vi "plot_functions.vi"() -> ()   [LabVIEW 2013]
doc: "opens a plot window and can access all the plot functions for testing"
uses:
  Classes/StatusLog/StatusLog.lvclass
  Classes/Plots/Plots.lvclass
  global variables.vi
  <vilib>/Utility/file.llb/Read From Spreadsheet File (string).vi
  MSEval/global_variables.vi
panel:
  in  "Combo Box":string(combo)="linear"
  in  "fit button":bool
  in  "data file":path=path "C:/Users/Thermo/Documents/GitHub/HelixMC/MSControl/test_vis/plot_data_he3.txt"
  in  "plot dataset button":bool
  in  "open plot button":bool
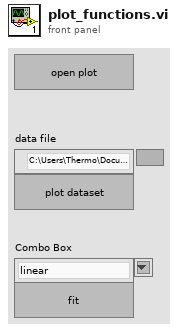
[diagram p1: front panel]
types:
  T1 = cluster{"log identifier":string, "active?":bool}[]
  T2 = cluster{"format string":string, "Variant":variant}
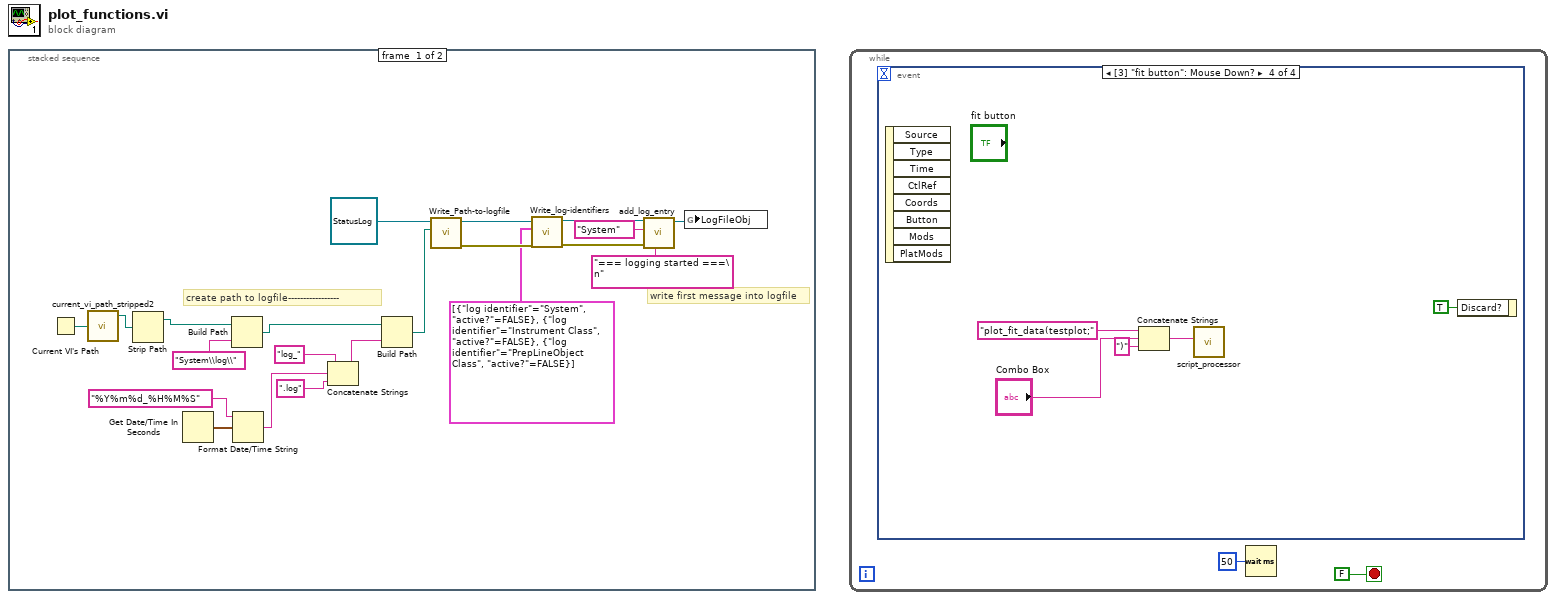
[diagram p0: block diagram]
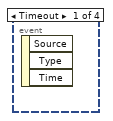
[diagram p2: hidden frame]
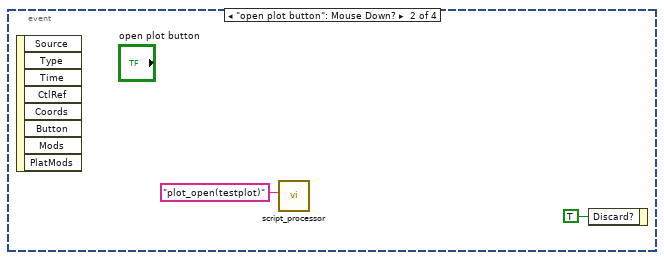
[diagram p3: hidden frame]
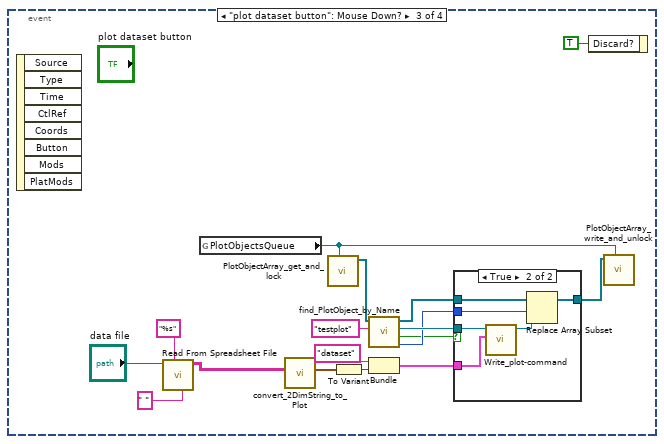
[diagram p4: hidden frame]
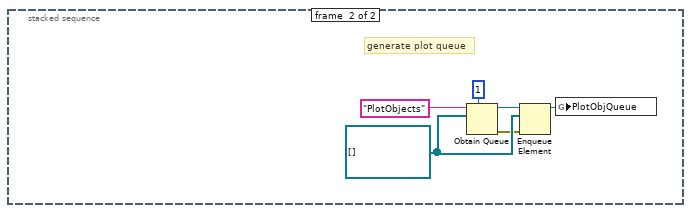
[diagram p6: hidden frame]
diagram:
  n1 = stacked-sequence {
    frame #0 {
      # "write first message into logfile"
      # "create path to logfile-----------------"
      n2 = Current VI's Path() -> (path=w4:path)
      n3 = call "current_vi_path_stripped2.vi"("current VI Path"=w4) -> ("current VI Path stripped out"=w2:path)  [unwired: 3 in, 1 out]
      n4 = Strip Path(path=w2) -> (stripped path=w1:path)  [unwired: 1 out]
      n5 = Get Date/Time In Seconds() -> (seconds since 1Jan1904=w19:timestamp)
      n6 = Build Path(base path=w1, name or relative path="System\\log\\") -> (appended path=w20:path)
      n7 = Format Date/Time String(time format string (%c)="%Y%m%d_%H%M%S", seconds (now)=w19) -> (date/time string=w15:string)  [unwired: 1 in]
      n8 = Concatenate Strings("log_" ("string"), w15, ".log" ("string")) -> (w17:string)
      n9 = Build Path(base path=w20, name or relative path=w17) -> (appended path=w16:path)
      n10 = call-dynamic "Write_Path-to-logfile.vi"("Path to logfile"=w16, "StatusLog in"=refnum<class "StatusLog.lvclass"> refnum ("StatusLog.lvclass")) -> ("error out"=w8:errorcluster, "StatusLog out"=w10:refnum<class "StatusLog.lvclass">)  [unwired: 8 in]
      n11 = call-dynamic "Write_log-identifiers.vi"("error in (no error)"=w8, "log identifiers"=T1 [{"log identifier"="System", "active?"=FALSE}, {"log identifier"="Instrument Class", "active?"=FALSE}, {"log identifier"="PrepLineObject Class", "active?"=FALSE}], "StatusLog in"=w10) -> ("error out"=w7:errorcluster, "StatusLog out"=w9:refnum<class "StatusLog.lvclass">)  [unwired: 7 in]
      n12 = call-dynamic "add_log_entry.vi"("new entry"="=== logging started ===\n", "error in (no error)"=w7, "log identifiers"="System", "StatusLog in"=w9) -> ("StatusLog out"=w11:refnum<class "StatusLog.lvclass">)  [unwired: 4 in, 1 out]
      n13 = global write "global variables.vi" "LogFileObj"(w11) -> ()
    }
    frame #1 {
      w24 = refnum<class "Plots.lvclass">[] [] ("PlotObjArray")
      # "generate plot queue"
      n14 = Obtain Queue(max queue size (-1, unlimited)=1, name (unnamed)="PlotObjects", element data type=w24) -> (queue out=w25:refnum<queue>, error out=w22:errorcluster)  [unwired: 2 in, 1 out]
      n15 = Enqueue Element(queue=w25, element=w24, error in (no error)=w22) -> (queue out=w23:refnum<queue>)  [unwired: 1 in, 2 out]
      n16 = global write "global variables.vi" "PlotObjQueue"(w23) -> ()
    }
  }
  n17 = while {
    stop <- FALSE stop-if-true
    n18 = event shown="[3] \"fit button\": Mouse Down?" {
      selector: _ -> [_ _ _ _]
      dyn-events: _ -> [_ _ _ _]
      timeout: _ -> [_ _ _ _]
      event Timeout {
        n19 = event-data() -> ()  [unwired: 1 in, 3 out]
      }
      event "open plot button": Mouse Down? {
        n20 = event-data() -> ()  [unwired: 1 in, 8 out]
        n21 = call "script_processor.vi"("command"="plot_open(testplot)") -> ()  [unwired: 10 in, 1 out]
        n22 = event-data("Discard?"=TRUE) -> ()  [unwired: 1 in, 1 out]
      }
      event "plot dataset button": Mouse Down? {
        n23 = event-data() -> ()  [unwired: 1 in, 8 out]
        n24 = call-poly <vilib>:"Read From Spreadsheet File.vi"("delimiter (\\t)"=" " ("delimiter (\\t)"), "format (%s)"="%s" ("format (%.3f)"), "file path (dialog if empty)"="data file") -> ("all rows"=w33:string[][])  [unwired: 4 in, 4 out]
        n25 = global read "global_variables.vi" "PlotObjectsQueue"() -> (w47:refnum<queue>)
        n26 = call "convert_2DimString_to_Plot.vi"("string data in"=w33) -> ("Plot Data"=w39:cluster{dbl, dbl, "flag":u8}[])  [unwired: 9 in, 1 out]
        n27 = call "PlotObjectArray_get_and_lock.vi"("External PlotObjQueue in"=w47) -> ("PlotObjects"=w46:refnum<class "Plots.lvclass">[])  [unwired: 9 in, 1 out]
        n28 = To Variant(anything=w39) -> (Variant=w40:variant)
        n29 = call "find_PlotObject_by_Name.vi"("Plot Name/ID"="testplot", "PlotObj Array in"=w46) -> ("index of Object in Array"=w44:i32, "found?"=w37:bool, "found PlotObj out"=w45:refnum<class "Plots.lvclass">, "PlotObj Array out"=w43:refnum<class "Plots.lvclass">[])  [unwired: 6 in]
        n30 = Bundle("format string"="dataset", "Variant"=w40) -> (w38:T2)  [unwired: 1 in]
        n31 = case shown="True" w37 {
          tunnel: w45 -> [_ w55]
          tunnel: w44 -> [_ w53]
          tunnel: w43 -> [w49 w52]
          tunnel: [w49 w51] -> w42
          tunnel: w38 -> [_ w50]
          frame False {
          }
          frame True {
            n32 = call-dynamic "Write_plot-command.vi"("plot command"=w50, "Plots in"=w55) -> ("Plots out"=w54:refnum<class "Plots.lvclass">)  [unwired: 8 in, 1 out]
            n33 = Replace Array Subset(array=w52, new element=w54, index=w53) -> (w51:refnum<class "Plots.lvclass">[])
          }
        }
        n34 = event-data("Discard?"=TRUE) -> ()  [unwired: 1 in, 1 out]
        n35 = call "PlotObjectArray_write_and_unlock.vi"("External PlotObjQueue in"=w47, "PlotObjects"=w42) -> ()  [unwired: 9 in, 1 out]
      }
      event "fit button": Mouse Down? {
        n36 = event-data() -> ()  [unwired: 1 in, 8 out]
        n37 = Concatenate Strings("plot_fit_data(testplot;" ("string"), "Combo Box", ")" ("string")) -> (w56:string)
        n38 = call "script_processor.vi"("command"=w56) -> ()  [unwired: 10 in, 1 out]
        n39 = event-data("Discard?"=TRUE) -> ()  [unwired: 1 in, 1 out]
      }
    }
    n40 = Wait (ms)(milliseconds to wait=u32 50) -> ()  [unwired: 1 out]
  }
